vi "Notifier References FGV.vi"(8 "error in":errorcluster, 11 "function":enum16{"obtain", "get", "release"}(ring)) -> (0 "error out":errorcluster, 3 "module notifiers":T1)   [LabVIEW 2017, in "myPAM.lvlib"]
uses:
  myPAM.lvlib
  Private TypeDefs/Module Notifiers.ctl
  Public TypeDefs/Current Position Data.ctl
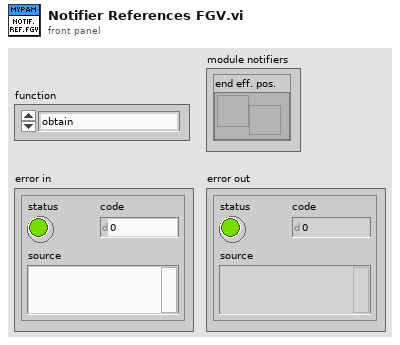
[diagram p1: front panel]
types:
  T1 = typedef "myPAM.lvlib/Module Notifiers.ctl" = cluster{"end eff. pos.":refnum<notifier>}
  T2 = typedef "myPAM.lvlib/Current Position Data.ctl" = cluster{"link 2 x (mm)":dbl, "link 2 y (mm)":dbl, "link 1 x (mm)":dbl, "link 1 y (mm)":dbl}
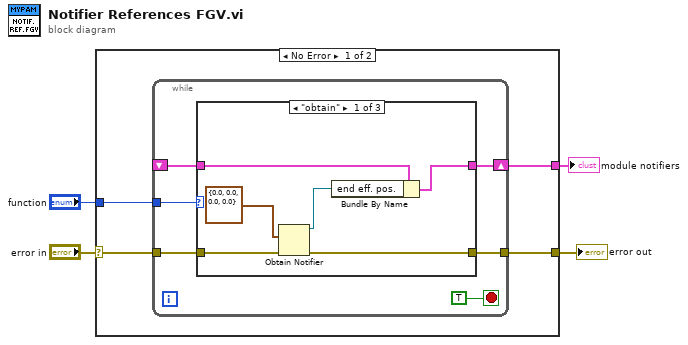
[diagram p0: block diagram]
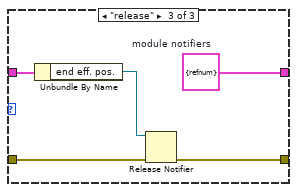
[diagram p3: hidden frame]
diagram:
  n1 = case shown="No Error" "error in" {
    selector: "error in" -> [w8 w28]
    tunnel: [w7 w28] -> w3
    tunnel: "function" -> [w6 _]
    tunnel: [w5 _] -> w1
    frame No Error {
      n2 = while {
        tunnel: w8 -> [w13]
        tunnel: [w12] -> w7
        tunnel: w6 -> [w11]
        shift-right: [w10] -> w5
        shift-left: _ -> [w9]
        stop <- TRUE stop-if-true
        n3 = case shown="\"obtain\"" w11 {
          tunnel: w13 -> [w20 w22 w27]
          tunnel: [w19 w22 w26] -> w12
          tunnel: [w17 w21 w25] -> w10
          tunnel: w9 -> [w18 w21 w24]
          frame "obtain" {
            n4 = Obtain Notifier(notification data type=T2 {"link 2 x (mm)"=0.0, "link 2 y (mm)"=0.0, "link 1 x (mm)"=0.0, "link 1 y (mm)"=0.0} ("End Effector Position"), error in (no error)=w20) -> (notifier out=w16:refnum<notifier>, error out=w19:errorcluster)  [unwired: 2 in, 1 out]
            n5 = Bundle By Name(cluster=w18, "end eff. pos."=w16) -> (w17:T1)
          }
          frame "get", Default {
          }
          frame "release" {
            w25 = T1 {"end eff. pos."=refnum}  # module notifiers
            n6 = Unbundle By Name(w24) -> ("end eff. pos."=w23:refnum<notifier>)
            n7 = Release Notifier(notifier=w23, error in (no error)=w27) -> (error out=w26:errorcluster)  [unwired: 1 in, 2 out]
          }
        }
      }
    }
    frame Error {
    }
  }
  "error out" <- w3
  "module notifiers" <- w1
